vi "RS485 CRC.vi"(9 "Data In":u8[](array[numeric])) -> (1 "Data+CRC":u8[](array[numeric]))   [LabVIEW 2014]
panel:
  # "VI Name: MB CRC-16.vi\nPurpose: Computes the CRC of a string.\nReentrant VI, because its caller is also reentrant."
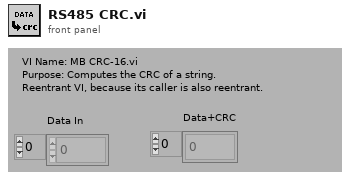
[diagram p1: front panel]
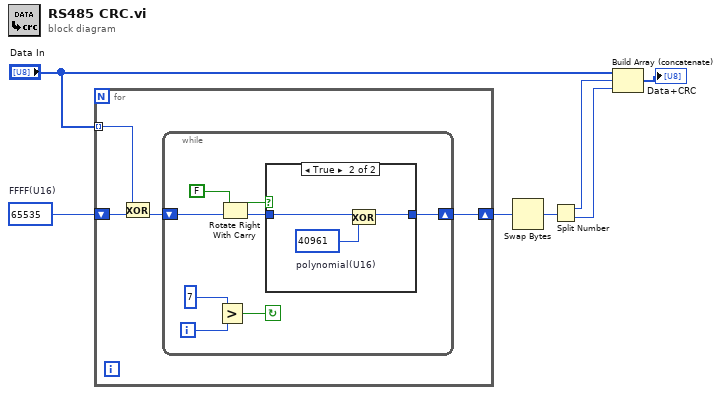
[diagram p0: block diagram]
diagram:
  w7 = u16 65535  # FFFF(U16)
  n1 = for {
    tunnel: "Data In" -> [w11] mode=indexing
    shift-right: [w8] -> w6
    shift-left: w7 -> [w10]
    n2 = Exclusive Or(1:w10, 2:w11) -> (0:w9:u16)
    n3 = while {
      shift-right: [w15] -> w8
      shift-left: w9 -> [w13]
      i -> [w14]
      stop <- w12 continue-if-true
      n4 = Greater?(x=7, y=w14) -> (0:w12:bool)
      n5 = Rotate Right With Carry(2:w13, 3:FALSE) -> (0:w16:u16, 1:w17:bool)
      n6 = case shown="True" w17 {
        tunnel: w16 -> [w20 w23]
        tunnel: [w20 w21] -> w15
        frame False {
        }
        frame True {
          w22 = u16 40961  # polynomial(U16)
          n7 = Exclusive Or(1:w22, 2:w23) -> (0:w21:u16)
        }
      }
    }
  }
  n8 = Swap Bytes(anything=w6) -> (byte swapped=w3:u16)
  n9 = Split Number(x=w3) -> (hi(x)=w1:u8, lo(x)=w2:u8)
  n10 = Build Array (concatenate)("Data In", w1, w2) -> (→"Data+CRC":u8[])
